vi "VCS Send CAN Frame.vi"(8 "error in (no error)":errorcluster, 9 "CAN frame":cluster{"cobId":u16, "length":u16, "data":u8[]}={"cobId"=0, "length"=0, "data"=[0, 0, 0, 0, 0, 0, 0, 0, 0, 0, 0, 0]} {"data" format="%x"}, 11 "keyHandle in":u32) -> (0 "error out":errorcluster, 3 "keyHandle out":u32)   [LabVIEW 2010]
doc: "<B>VCS Send CAN Frame</B> sends a general CAN Frame to the CAN bus."
uses:
  Resources/EposCmd.dll
  Resources/EposCmd64.dll
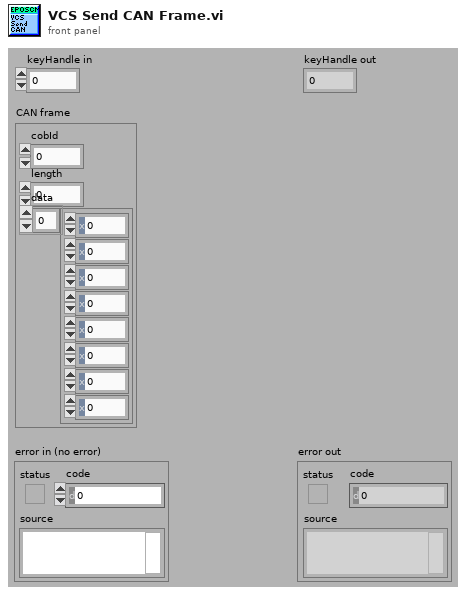
[diagram p1: front panel]
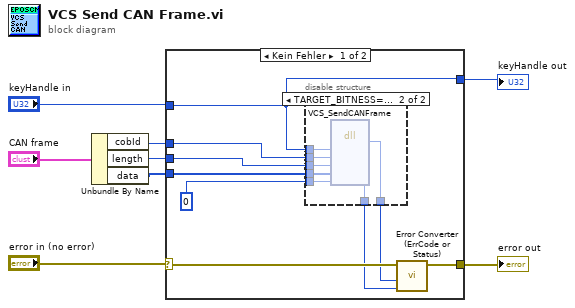
[diagram p0: block diagram]
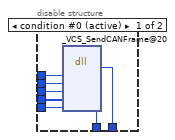
[diagram p2: hidden frame]
diagram:
  n1 = Unbundle By Name("CAN frame") -> ("cobId"=w2:u16, "length"=w1:u16, "data"=w3:u8[])
  n2 = case shown="Kein Fehler" "error in (no error)" {
    selector: "error in (no error)" -> [w17 w33]
    tunnel: [w16 w33] -> w7
    tunnel: "keyHandle in" -> [w13 w32]
    tunnel: [w13 w32] -> w5
    tunnel: w3 -> [w11 _]
    tunnel: w2 -> [w10 _]
    tunnel: w1 -> [w9 _]
    frame No Error {
      n3 = disable-structure shown="TARGET_BITNESS==64" {
        disable-tunnel: [w24 w31] -> w15
        disable-tunnel: u32 0 ("pErrorCode") -> [w23 w30]
        disable-tunnel: w13 -> [w22 w29]
        disable-tunnel: [w21 w28] -> w12
        disable-tunnel: w11 -> [w20 w27]
        disable-tunnel: w10 -> [w19 w26]
        disable-tunnel: w9 -> [w18 w25]
        frame condition #0 (active) {
          n4 = dll-call lib="C:/Sources/LabView/maxon EPOS/Resources/EposCmd.*" fn="_VCS_SendCANFrame@20"("KeyHandle"=w22, "CobID"=w19, "Length"=w18, "pData"=w20, "pErrorCode"=w23) -> (w21:i32, "pErrorCode"=w24:u32)  [unwired: 7 in, 2 out]
        }
        frame condition #1 {
          n5 = dll-call lib="C:/setup/Resources/EposCmd64.*" fn="VCS_SendCANFrame" ("EposCmd.dll:_VCS_SendCANFrame@20")("KeyHandle"=w29, "CobID"=w26, "Length"=w25, "pData"=w27, "pErrorCode"=w30) -> ("Rückgabetyp"=w28:i32, "pErrorCode"=w31:u32)  [unwired: 7 in, 2 out]
        }
      }
      n6 = call "Error Converter (ErrCode or Status).vi"("error code"=w15, "return type"=w12, "error in (no error)"=w17) -> ("error out"=w16:errorcluster)  [unwired: 7 in]
    }
    frame Error {
    }
  }
  "error out" <- w7
  "keyHandle out" <- w5
